vi "DETUpdate-Com-exec.vi"(8 "error in (no error)":errorcluster, 10 "data":variant, 11 "Detector in":refnum<class "Detector.lvclass">) -> (0 "error out":errorcluster, 2 "Cooler status":bool, 3 "Detector out":refnum<class "Detector.lvclass">)   [LabVIEW 2020, in "Detector.lvclass"]
uses:
  Detector.lvclass
  C:/dev/TRANCON/Classes/GeneralFunctionality/GeneralFunctionality.lvclass
  GeneralFunctionality/GeneralFunctionality.lvclass/GeneralFunctionality.ctl
  Detector.lvclass/Detector.ctl
  GeneralFunctionality/GeneralFunctionality.lvclass
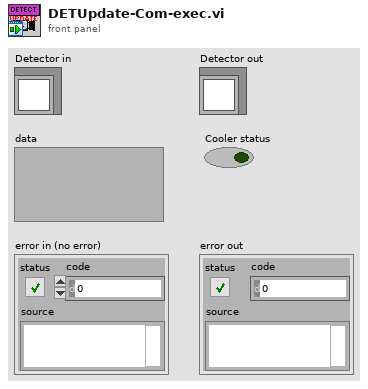
[diagram p1: front panel]
types:
  T1 = enum8{"Enabled", "Disabled", "Disabled and Grayed Out"}
  T2 = typedef "Control-Client.lvclass/Controls-refs_CLIENT.ctl" = cluster{"ON/OFF Cool":refnum<vi>, "Save spectra":refnum<vi>, "Read detector":refnum<vi>, "# scans":refnum<vi>, "BG-level":refnum<vi>, "Set T":refnum<vi>, "Termometer":refnum<vi>, "Spectra":refnum<vi>, "Error Meter_ref":refnum<vi>, "OD graph":refnum<vi>, "from_pixel":refnum<vi>, "to_pixel":refnum<vi>, "threshold_ref_channel":refnum<vi>, "value":refnum<vi>, "python session":refnum<vi>, "ref h5_file":T3, "distance":refnum<vi>}
  T3 = typedef "hid_t.ctl" = i64
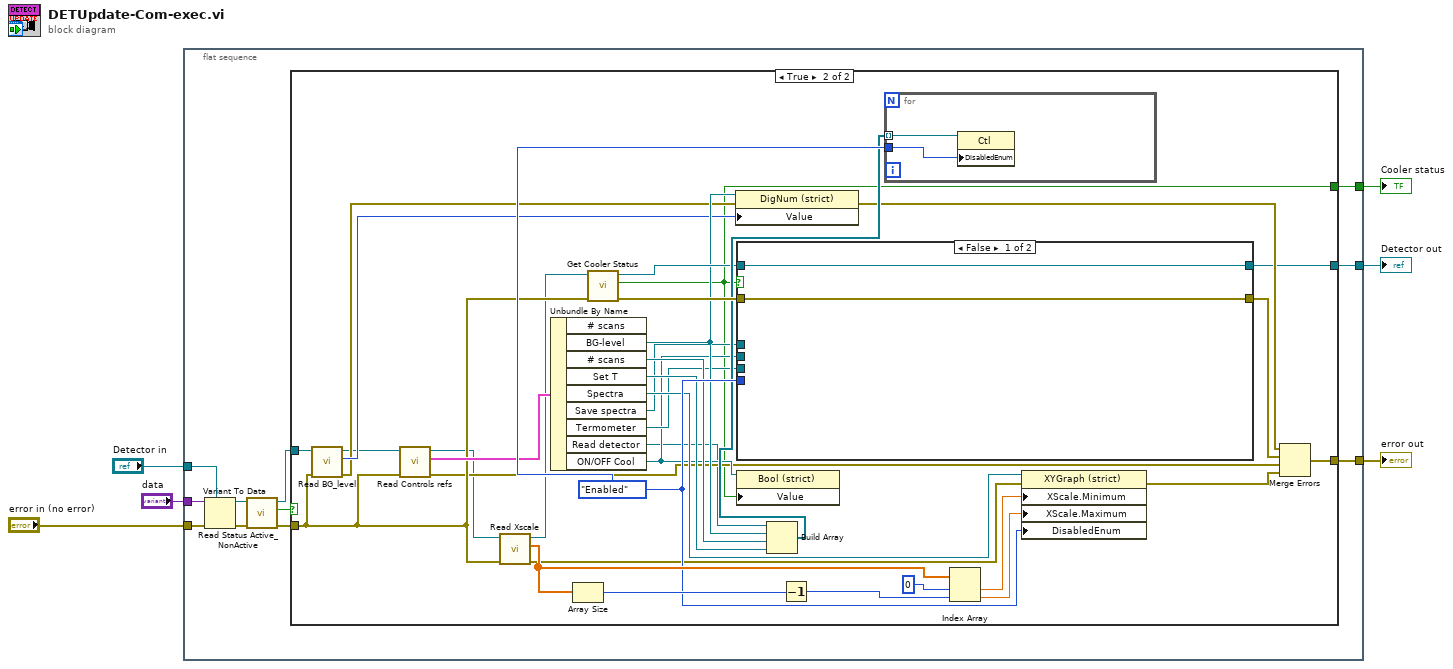
[diagram p0: block diagram]
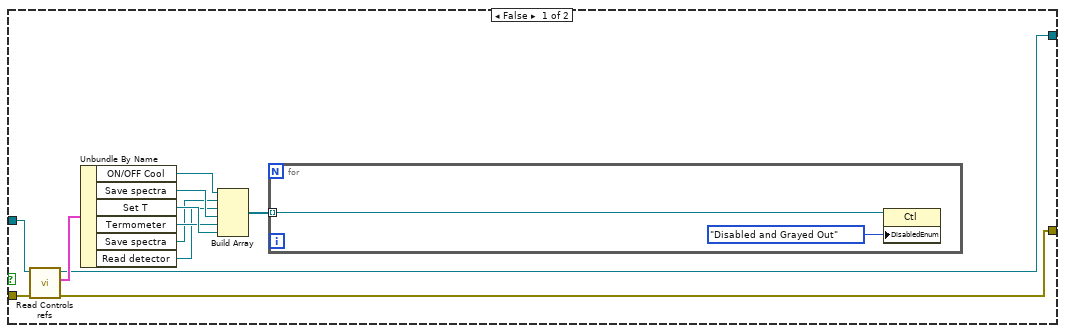
[diagram p2: hidden frame]
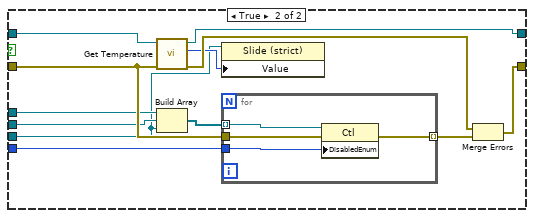
[diagram p3: hidden frame]
diagram:
  n1 = flat-sequence {
    tunnel: "Detector in" -> [w17]
    tunnel: "data" -> [w16]
    tunnel: "error in (no error)" -> [w15]
    tunnel: [w7] -> w4
    tunnel: [w9] -> w5
    tunnel: [w8] -> w6
    frame #0 {
      n2 = Variant To Data(error in=w15, type=w17, Variant=w16) -> (data=w14:refnum<class "Detector.lvclass">, error out=w13:errorcluster)
      n3 = call "Read Status Active_NonActive.vi"("error in (no error)"=w13, "GeneralFunctionality in"=w14) -> ("error out"=w12:errorcluster, "Status Active/NonActive"=w11:bool, "GeneralFunctionality out"=w10:refnum<class "Detector.lvclass">)  [unwired: 7 in]
      n4 = case shown="True" w11 {
        tunnel: w12 -> [w19 w43]
        tunnel: w10 -> [w28 w36]
        tunnel: [w18 w55] -> w8
        tunnel: [_ w38] -> w9
        tunnel: [w20 w32] -> w7
        frame False {
          n5 = call "Read Controls refs.vi"("error in (no error)"=w19, "Detector in"=w28) -> ("error out"=w18:errorcluster, "Controls refs"=w27:T2, "Detector out"=w20:refnum<class "Detector.lvclass">)  [unwired: 7 in]
          n6 = Unbundle By Name(w27) -> ("ON/OFF Cool"=w26:refnum<vi>, "Save spectra"=w25:refnum<vi>, "Set T"=w24:refnum<vi>, "Termometer"=w23:refnum<vi>, "Save spectra"=w22:refnum<vi>, "Read detector"=w21:refnum<vi>)
          n7 = Build Array(w26, w22, w21, w25, w23, w24) -> (w29:refnum<vi>[])
          n8 = for {
            tunnel: w29 -> [w30] mode=indexing
            n9 = property class="Ctl"(reference=w30, "DisabledEnum"=T1."Disabled and Grayed Out" ("Désactivé")) -> ()  [unwired: 1 in, 2 out]
          }
        }
        frame True {
          w59 = T1."Enabled" ("Désactivé")
          n10 = call-dynamic "Read BG_level.vi"("error in (no error)"=w43, "Detector in"=w36) -> ("error out"=w42:errorcluster, "BG_level"=w48:i32, "Detector out"=w35:refnum<class "Detector.lvclass">)  [unwired: 7 in]
          n11 = call "Read Controls refs.vi"("error in (no error)"=w43, "Detector in"=w35) -> ("error out"=w39:errorcluster, "Controls refs"=w52:T2, "Detector out"=w34:refnum<class "Detector.lvclass">)  [unwired: 7 in]
          n12 = call "Read Xscale.vi"("error in (no error)"=w43, "Detector en entrée"=w34) -> ("error out"=w58:errorcluster, "Xscale"=w65:dbl[], "Detector en sortie"=w33:refnum<class "Detector.lvclass">)  [unwired: 7 in]
          n13 = Unbundle By Name(w52) -> ("BG-level"=w49:refnum<vi>, "# scans"=w51:refnum<vi>, "Set T"=w50:refnum<vi>, "Spectra"=w47:refnum<vi>, "Save spectra"=w46:refnum<vi>, "Termometer"=w45:refnum<vi>, "Read detector"=w37:refnum<vi>, "ON/OFF Cool"=w44:refnum<vi>)  [unwired: 1 out]
          n14 = Array Size(array=w65) -> (size(s)=w64:i32)
          n15 = call "Get Cooler Status.vi"("error in (no error)"=w43, "Detector in"=w33) -> ("error out"=w57:errorcluster, "Cooler status"=w38:bool, "Detector out"=w53:refnum<class "Detector.lvclass">)  [unwired: 7 in]
          n16 = property class="DigNum (strict)"(reference=w49, error in=w42, "Value"=w48) -> (error out=w41:errorcluster)  [unwired: 1 out]
          n17 = case shown="False" w38 {
            tunnel: w59 -> [_ w80]
            tunnel: w57 -> [w69 w76]
            tunnel: [w69 w78] -> w56
            tunnel: w53 -> [w68 w77]
            tunnel: w46 -> [_ w74]
            tunnel: w45 -> [_ w71]
            tunnel: w44 -> [_ w72]
            tunnel: [w68 w70] -> w32
            frame False {
            }
            frame True {
              n18 = call-dynamic "Get Temperature.vi"("error in (no error)"=w76, "Detector in"=w77) -> ("error out"=w75:errorcluster, "Temperature"=w73:i32, "Detector out"=w70:refnum<class "Detector.lvclass">)  [unwired: 7 in]
              n19 = Build Array(w74, w72, w71) -> (w81:refnum<vi>[])
              n20 = property class="Slide (strict)"(reference=w71, "Value"=w73) -> ()  [unwired: 1 in, 2 out]
              n21 = for {
                tunnel: w81 -> [w85] mode=indexing
                tunnel: w80 -> [w84]
                tunnel: w76 -> [w83]
                tunnel: [w82] -> w79 mode=indexing
                n22 = property class="Ctl"(reference=w85, error in=w83, "DisabledEnum"=w84) -> (error out=w82:errorcluster)  [unwired: 1 out]
              }
              n23 = Merge Errors(w75, w79) -> (w78:errorcluster)
            }
          }
          n24 = property class="Bool (strict)"(reference=w44, "Value"=w38) -> ()  [unwired: 1 in, 2 out]
          n25 = Build Array(w37, w49, w51, w50) -> (w54:refnum<vi>[])
          n26 = Decrement(x=w64) -> (x-1=w60:i32)
          n27 = for {
            tunnel: w59 -> [w67]
            tunnel: w54 -> [w66] mode=indexing
            n28 = property class="Ctl"(reference=w66, "DisabledEnum"=w67) -> ()  [unwired: 1 in, 2 out]
          }
          n29 = Index Array(array=w65, index #1=0 ("indice"), index #2=w60) -> (element #1=w62:dbl, element #2=w61:dbl)
          n30 = property class="XYGraph (strict)"(reference=w47, error in=w58, "XScale.Minimum"=w62, "XScale.Maximum"=w61, "DisabledEnum"=w59) -> (error out=w40:errorcluster)  [unwired: 1 out]
          n31 = Merge Errors(w41, w56, w39, w40) -> (w55:errorcluster)
        }
      }
    }
  }
  "error out" <- w6
  "Cooler status" <- w5
  "Detector out" <- w4
